vi "File Writing.vi"(6 "Filename":string, 7 "File extension":string, 9 "?":bool, 10 "Array":dbl[](array[numeric]), 11 "Path":path) -> (0 "error out":errorcluster, 2 "WRITING TO FILE":bool, 3 "Full filepath":string)   [LabVIEW 2020]
uses:
  <vilib>/Utility/file.llb/Write Delimited Spreadsheet (DBL).vi
  <vilib>/Analysis/Matrix/NI_Matrix.lvlib
  <vilib>/Analysis/Matrix/Numeric/Conversions/Array To Matrix - RA.vi
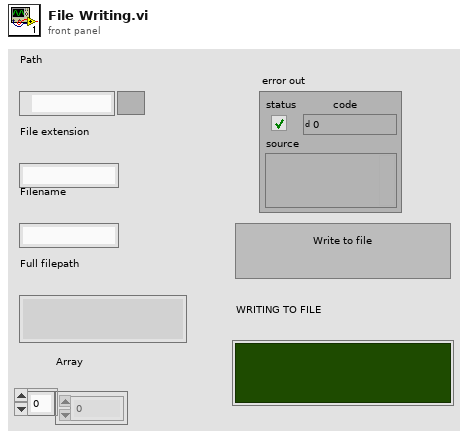
[diagram p1: front panel]
types:
  T1 = typedef "NI_Matrix.lvlib/RealMatrix.ctl" = dbl[][]
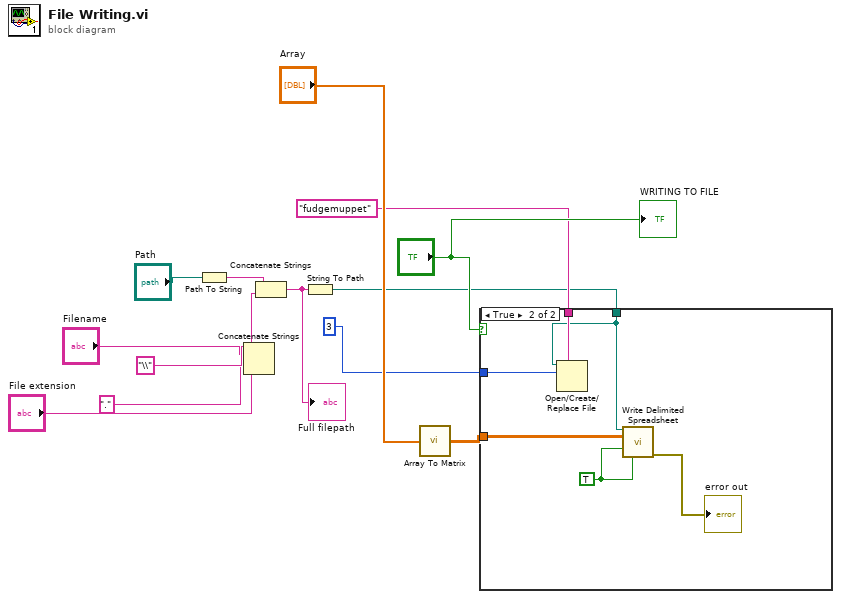
[diagram p0: block diagram]
diagram:
  n1 = Path To String(path="Path") -> (string=w2:string)
  n2 = Concatenate Strings("\\", "Filename", ".", "File extension") -> (w3:string)
  n3 = Concatenate Strings(w2, w3) -> (w4:string)
  "Full filepath" <- w4
  n4 = String To Path(string=w4) -> (path=w9:path)
  n5 = call-poly <vilib>:"Array To Matrix.vi"("Real 1D Array"="Array") -> ("Real Matrix (Column Vector)"=w13:T1)
  n6 = case shown="True" "?" {
    tunnel: w9 -> [_ w18]
    tunnel: w13 -> [_ w15]
    tunnel: "fudgemuppet" -> [_ w20]
    tunnel: 3 -> [_ w19]
    frame False {
    }
    frame True {
      w16 = TRUE
      n7 = Open/Create/Replace File(file path (use dialog)=w18, prompt=w20, operation (0:open)=w19) -> ()  [unwired: 3 in, 3 out]
      n8 = call-poly <vilib>:"Write Delimited Spreadsheet.vi"("file path (dialog if empty)"=w18, "2D data"=w15, "append to file? (new file:F)"=w16, "transpose? (no:F)"=w16) -> ("error out"=→"error out":errorcluster)  [unwired: 10 in, 1 out]
    }
  }
  "WRITING TO FILE" <- "?"
